vi "Pressure.vi"(0 "VISA resource name":refnum<visa-resource-name>, 1 "baud rate (9600)":u32=9600, 2 "data bits (8)":u16=8 min=5 max=8 step=1, 3 "parity (0:none)":dbl, 4 "stop bits (10: 1 bit)":u16=10, 5 "flow control (0:none)":dbl, 6 "Recieve Data":bool, 7 "termination char\n(0xA = '\\n' = LF)":u8=13 format="%.0x") -> (13 "VISA resource name out":refnum<visa-resource-name>, 14 "output cluster":cluster{dbl, dbl, dbl}, 15 "output array":string[](array[string]), 16 "Response G1":string, 17 "Response G2":string, 18 "Response G3":string, 19 "error out":errorcluster)   [LabVIEW 2019]
uses:
  <vilib>/Instr/_visa.llb/VISA Configure Serial Port (Instr).vi
panel:
  out "bytes read 3":u32
  out "bytes read 2":u32
  out "bytes read":u32
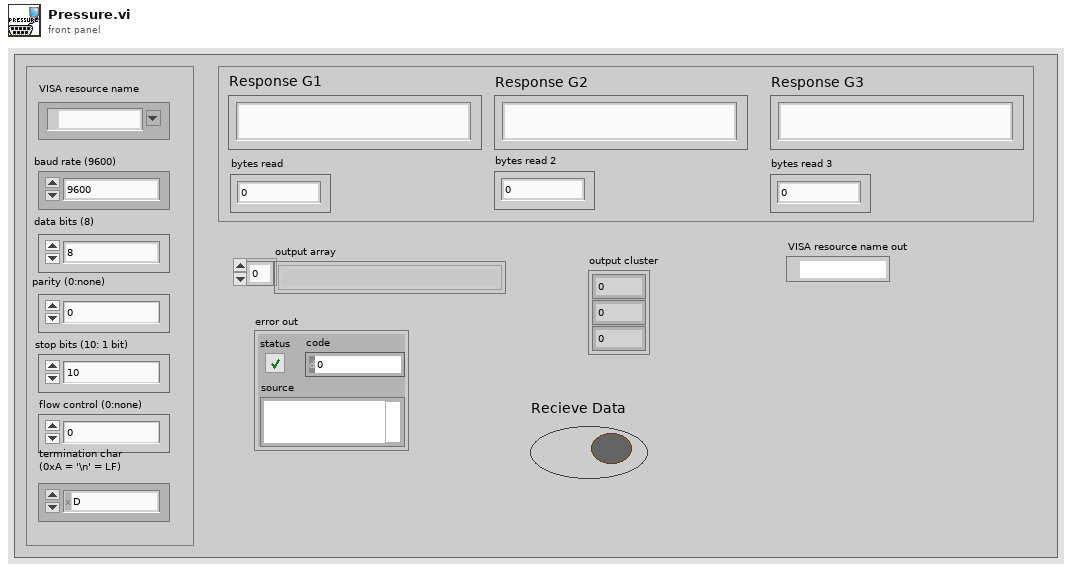
[diagram p1: front panel]
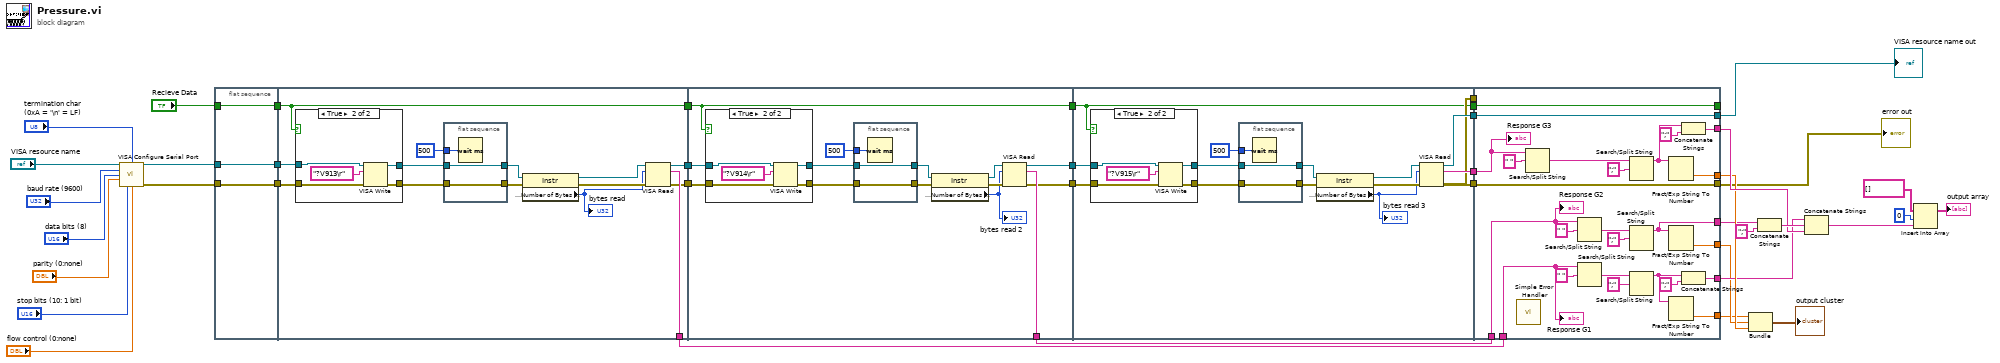
[diagram p0: block diagram]
diagram:
  n1 = call-poly "VISA Configure Serial Port"("VISA resource name"="VISA resource name", "termination char\n(0xA = '\\n' = LF)"="termination char\n(0xA = '\\n' = LF)", "baud rate (9600)"="baud rate (9600)", "data bits (8)"="data bits (8)", "parity (0:none)"="parity (0:none)", "stop bits (10: 1 bit)"="stop bits (10: 1 bit)", "flow control (0:none)"="flow control (0:none)") -> ("VISA resource name out"=w19:refnum<visa-resource-name>, "error out"=w18:errorcluster)  [unwired: 3 in, 4 out]
  n2 = flat-sequence {
    tunnel: w19 -> [w42]
    tunnel: w18 -> [w43]
    tunnel: "Recieve Data" -> [w44]
    tunnel: [w44] -> w34
    tunnel: [w43] -> w33
    tunnel: [w42] -> w32
    tunnel: [w48] -> w7
    tunnel: [w47] -> w31
    tunnel: [w46] -> w30
    tunnel: [w45] -> w29
    tunnel: w34 -> [w45]
    tunnel: w33 -> [w53]
    tunnel: w32 -> [w52]
    tunnel: w31 -> [w77]
    tunnel: w30 -> [w76]
    tunnel: [w72] -> w8
    tunnel: [w70] -> w28
    tunnel: [w71] -> w27
    tunnel: w29 -> [w69]
    tunnel: [w69] -> w26
    tunnel: w28 -> [w103]
    tunnel: w27 -> [w102]
    tunnel: w26 -> [w93]
    tunnel: [w94] -> w15
    tunnel: [w96] -> w14
    tunnel: [w95] -> w13
    tunnel: [w94] -> w12
    tunnel: [w93] -> w11
    tunnel: [w139] -> _
    tunnel: [w140] -> w1
    tunnel: w15 -> [_]
    tunnel: w14 -> [w117]
    tunnel: w13 -> [w141]
    tunnel: w12 -> [w140]
    tunnel: w11 -> [w139]
    tunnel: [w133] -> w10
    tunnel: [w132] -> w9
    tunnel: w8 -> [w125]
    tunnel: w7 -> [w122]
    tunnel: [w121] -> w6
    tunnel: [w120] -> w5
    tunnel: [w119] -> w4
    tunnel: [w118] -> w3
    tunnel: [w117] -> w2
    frame #0 {
    }
    frame #1 {
      n3 = case shown="True" w45 {
        tunnel: w53 -> [w59 w65]
        tunnel: w52 -> [w60 w64]
        tunnel: [w59 w63] -> w51
        tunnel: [w60 w61] -> w50
        frame False {
        }
        frame True {
          n4 = VISA Write(VISA resource name=w64, write buffer="?V913\r" ("Command"), error in (no error)=w65) -> (VISA resource name out=w61:refnum<visa-resource-name>, error out=w63:errorcluster)  [unwired: 1 out]
        }
      }
      n5 = flat-sequence {
        tunnel: w51 -> [w67]
        tunnel: [w67] -> w58
        tunnel: u32 500 ("delay before read (ms)") -> [w68]
        tunnel: w50 -> [w66]
        tunnel: [w66] -> w49
        frame #0 {
          n6 = Wait (ms)(milliseconds to wait=w68) -> ()  [unwired: 1 out]
        }
      }
      n7 = property class="Instr"(reference=w49, error in=w58) -> (reference out=w56:refnum<visa-resource-name>, error out=w55:errorcluster, "Serial Settings:Number of Bytes at Serial Port"=w54:u32)
      "bytes read" <- w54
      n8 = VISA Read(VISA resource name=w56, byte count=w54, error in (no error)=w55) -> (VISA resource name out=w47:refnum<visa-resource-name>, read buffer=w48:string, error out=w46:errorcluster)  [unwired: 1 out]
    }
    frame #2 {
      n9 = case shown="True" w69 {
        tunnel: w77 -> [w84 w88]
        tunnel: w76 -> [w83 w87]
        tunnel: [w84 w86] -> w75
        tunnel: [w83 w85] -> w74
        frame False {
        }
        frame True {
          n10 = VISA Write(VISA resource name=w88, write buffer="?V914\r" ("Command"), error in (no error)=w87) -> (VISA resource name out=w86:refnum<visa-resource-name>, error out=w85:errorcluster)  [unwired: 1 out]
        }
      }
      n11 = flat-sequence {
        tunnel: w74 -> [w91]
        tunnel: [w91] -> w73
        tunnel: u32 500 ("delay before read (ms)") -> [w92]
        tunnel: w75 -> [w90]
        tunnel: [w90] -> w79
        frame #0 {
          n12 = Wait (ms)(milliseconds to wait=w92) -> ()  [unwired: 1 out]
        }
      }
      n13 = property class="Instr"(reference=w79, error in=w73) -> (reference out=w82:refnum<visa-resource-name>, error out=w81:errorcluster, "Serial Settings:Number of Bytes at Serial Port"=w80:u32)
      "bytes read 2" <- w80
      n14 = VISA Read(VISA resource name=w82, byte count=w80, error in (no error)=w81) -> (VISA resource name out=w71:refnum<visa-resource-name>, read buffer=w72:string, error out=w70:errorcluster)  [unwired: 1 out]
    }
    frame #3 {
      n15 = case shown="True" w93 {
        tunnel: w103 -> [w107 w112]
        tunnel: w102 -> [w108 w111]
        tunnel: [w107 w110] -> w100
        tunnel: [w108 w109] -> w99
        frame False {
        }
        frame True {
          n16 = VISA Write(VISA resource name=w111, write buffer="?V915\r" ("Command"), error in (no error)=w112) -> (VISA resource name out=w109:refnum<visa-resource-name>, error out=w110:errorcluster)  [unwired: 1 out]
        }
      }
      n17 = flat-sequence {
        tunnel: u32 500 ("delay before read (ms)") -> [w116]
        tunnel: w100 -> [w115]
        tunnel: w99 -> [w114]
        tunnel: [w115] -> w98
        tunnel: [w114] -> w97
        frame #0 {
          n18 = Wait (ms)(milliseconds to wait=w116) -> ()  [unwired: 1 out]
        }
      }
      n19 = property class="Instr"(reference=w97, error in=w98) -> (reference out=w106:refnum<visa-resource-name>, error out=w105:errorcluster, "Serial Settings:Number of Bytes at Serial Port"=w104:u32)
      "bytes read 3" <- w104
      n20 = VISA Read(VISA resource name=w106, byte count=w104, error in (no error)=w105) -> (VISA resource name out=w96:refnum<visa-resource-name>, read buffer=w95:string, error out=w94:errorcluster)  [unwired: 1 out]
    }
    frame #4 {
      n21 = call <vilib>:"Simple Error Handler.vi"() -> ()  [unwired: 2 in, 8 out]
      n22 = Search/Split String(string=w141, search string/char (-)=" ") -> (match + rest of string=w138:string)  [unwired: 1 in, 2 out]
      n23 = Search/Split String(string=w125, search string/char (-)=" ") -> (match + rest of string=w130:string)  [unwired: 1 in, 2 out]
      n24 = Search/Split String(string=w122, search string/char (-)=" ") -> (match + rest of string=w131:string)  [unwired: 1 in, 2 out]
      n25 = Search/Split String(string=w138, search string/char (-)=";") -> (substring before match=w137:string)  [unwired: 1 in, 2 out]
      n26 = Search/Split String(string=w130, search string/char (-)=";") -> (substring before match=w119:string)  [unwired: 1 in, 2 out]
      n27 = Search/Split String(string=w131, search string/char (-)=";") -> (substring before match=w129:string)  [unwired: 1 in, 2 out]
      n28 = Fract/Exp String To Number(string=w137) -> (number=w132:dbl)  [unwired: 3 in, 1 out]
      n29 = Fract/Exp String To Number(string=w119) -> (number=w120:dbl)  [unwired: 3 in, 1 out]
      n30 = Fract/Exp String To Number(string=w129) -> (number=w118:dbl)  [unwired: 3 in, 1 out]
      n31 = Concatenate Strings(w137, ";" ("string")) -> (w133:string)
      n32 = Concatenate Strings(w129, ";" ("string")) -> (w121:string)
      "Response G3" <- w141
      "Response G1" <- w122
      "Response G2" <- w125
    }
  }
  n33 = Bundle(w3, w5, w9) -> (→"output cluster":cluster{dbl, dbl, dbl})  [unwired: 1 in]
  n34 = Concatenate Strings(w4, ";" ("string")) -> (w24:string)
  n35 = Concatenate Strings(w6, w24, w10) -> (w25:string)
  n36 = Insert Into Array(array=string[] [], index=0, new element=w25) -> (→"output array":string[])
  "error out" <- w1
  "VISA resource name out" <- w2
